vi "Configure Baud Rate.vi"(8 "error in (no error)":errorcluster, 10 "Baud Rate (3: 57600)":u16(ring)=3 format="%x" items=["4800", "9600", "14400", "19200", "38400", "57600", "115200"], 11 "VISA resource name":refnum<visa-resource-name>) -> (0 "error out":errorcluster, 3 "VISA resource name out":refnum<visa-resource-name>)   [LabVIEW 2011, in "Ocean Server OS4000.lvlib"]
doc: "Set new baud rate change takes effect after power cycle"
uses:
  Ocean Server OS4000.lvlib
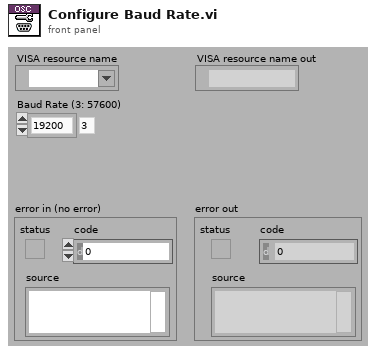
[diagram p1: front panel]
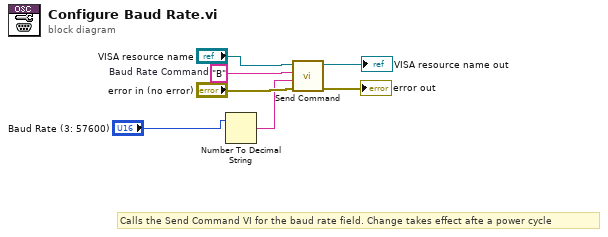
[diagram p0: block diagram]
diagram:
  w6 = "B"  # Baud Rate Command
  # "Calls the Send Command VI for the baud rate field. Change takes effect afte a power cycle"
  n1 = Number To Decimal String(number="Baud Rate (3: 57600)") -> (decimal integer string=w4:string)  [unwired: 1 in]
  n2 = call "Send Command.vi"("error in (no error)"="error in (no error)", "Value"=w4, "Message"=w6, "VISA resource name"="VISA resource name") -> ("error out"=→"error out":errorcluster, "VISA resource out"=→"VISA resource name out":refnum<visa-resource-name>)  [unwired: 6 in]
